vi "GetBacklogFiles.vi"(7 "LabVIEW Web Service Request":refnum<class "Web Request.lvclass">) -> ()   [LabVIEW 2017]
uses:
  <vilib>/wsapi/Web Request.lvclass
  <vilib>/addons/InsightCM/Utilities/GlobalConfiguration/GlobalConfiguration.lvlib
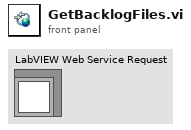
[diagram p1: front panel]
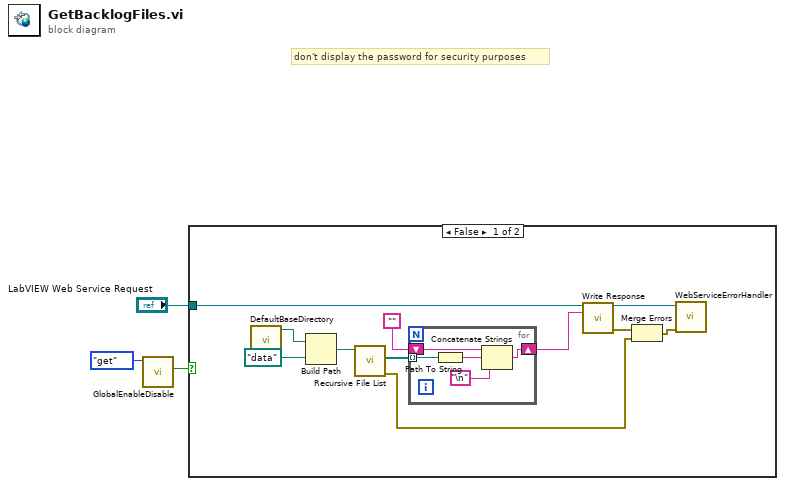
[diagram p0: block diagram]
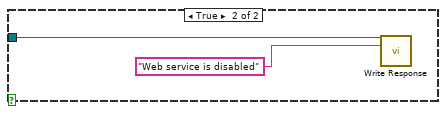
[diagram p2: hidden frame]
diagram:
  # "don't display the password for security purposes"
  n1 = call "GlobalEnableDisable.vi"("action"=enum16{"init", "set", "get"}."get") -> ("DisableDeviceWebService"=w1:bool)  [unwired: 10 in]
  n2 = case shown="False" w1 {
    tunnel: "LabVIEW Web Service Request" -> [w14 w20]
    frame False {
      n3 = call <vilib>:"DefaultBaseDirectory.vi"() -> ("base directory"=w9:path)  [unwired: 11 in]
      n4 = Build Path(base path=w9, name or relative path=path "data" ("base directory")) -> (appended path=w6:path)
      n5 = call <vilib>:"Recursive File List.vi"("Folder Path"=w6) -> ("error out"=w5:errorcluster, "All Files in Dir"=w7:path[])  [unwired: 6 in, 3 out]
      n6 = for {
        tunnel: w7 -> [w19] mode=indexing
        shift-right: [w17] -> w4
        shift-left: "" -> [w16]
        n7 = Path To String(path=w19) -> (string=w18:string)
        n8 = Concatenate Strings(w16, w18, "\n") -> (w17:string)
      }
      n9 = call <vilib>:"Write Response.vi"("LabVIEW Web Service Request"=w14, "response string"=w4) -> ("LabVIEW Web Service Request out"=w13:refnum<class "Web Request.lvclass">, "error out"=w12:errorcluster)  [unwired: 12 in]
      n10 = Merge Errors(w12, w5) -> (w11:errorcluster)
      n11 = call "WebServiceErrorHandler.vi"("LabVIEW Web Service Request"=w13, "error in (no error)"=w11) -> ()  [unwired: 12 in, 2 out]
    }
    frame True {
      n12 = call <vilib>:"Write Response.vi"("LabVIEW Web Service Request"=w20, "response string"="Web service is disabled") -> ()  [unwired: 12 in, 2 out]
    }
  }
